vi "DrawOrange.vi"(9 "Expression":string, 11 "String in":refnum<vi>) -> (3 "String out":refnum<vi>)   [LabVIEW 2016, in "Code.xctl"]
uses:
  <userlib>/MicroPython/VIs/ColorText/Code.xctl
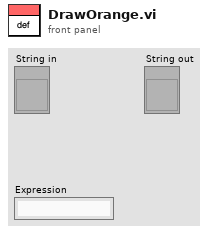
[diagram p1: front panel]
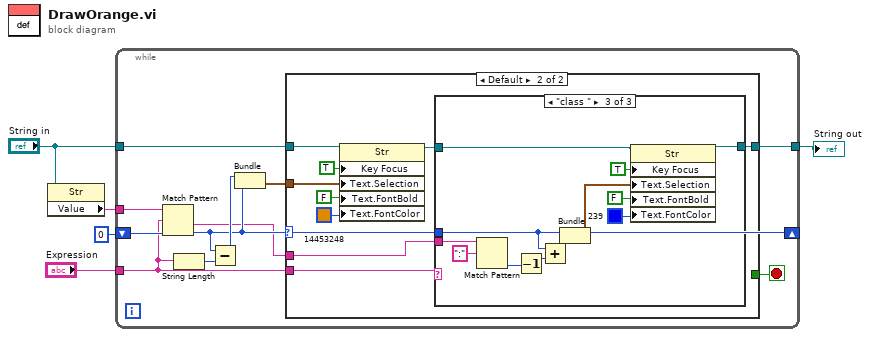
[diagram p0: block diagram]
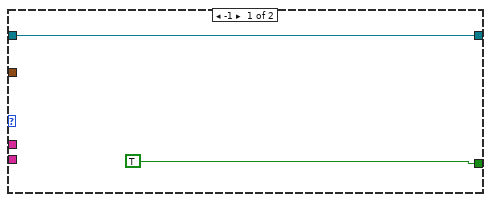
[diagram p2: hidden frame]
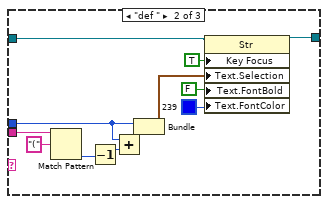
[diagram p4: hidden frame]
diagram:
  n1 = property on="Property Node" class="Str"(reference="String in") -> ("Value"=w1:string)  [unwired: 1 in, 2 out]
  n2 = while {
    tunnel: "String in" -> [w16]
    shift-right: [w9] -> _
    shift-left: 0 -> [w14]
    tunnel: w1 -> [w15]
    tunnel: [w10] -> w4
    tunnel: "Expression" -> [w7]
    stop <- w8 stop-if-true
    n3 = Match Pattern(string=w15, regular expression=w7, offset (0)=w14) -> (after substring=w6:string, offset past match=w9:i32)  [unwired: 2 out]
    n4 = String Length(string=w7) -> (length=w13:i32)
    n5 = Subtract(x=w9, y=w13) -> (x-y=w12:i32)
    n6 = Bundle(w12, "offset past match"=w9) -> (w11:cluster{i32, "offset past match":i32})  [unwired: 1 in]
    n7 = case shown="Default" w9 {
      selector: w9 -> [_ w21]
      tunnel: w16 -> [w18 w25]
      tunnel: w11 -> [_ w24]
      tunnel: [w18 w22] -> w10
      tunnel: [TRUE _] -> w8
      tunnel: w7 -> [_ w20]
      tunnel: w6 -> [_ w19]
      frame -1 {
      }
      frame Default {
        n8 = property on="Property Node" class="Str"(reference=w25, "Key Focus"=TRUE, "Text.Selection"=w24, "Text.FontBold"=FALSE ("Text.Font:Bold"), "Text.FontColor"=u32 14453248 ("Text.Text Colors:Text Color")) -> (reference out=w23:refnum<vi>)  [unwired: 1 in, 1 out]
        n9 = case shown="\"class \"" w20 {
          tunnel: w23 -> [w29 w38 w50]
          tunnel: [w29 w37 w49] -> w22
          tunnel: w21 -> [_ w34 w46]
          tunnel: w19 -> [_ w32 w44]
          frame Default {
          }
          frame "def " {
            n10 = Match Pattern(string=w32, regular expression="(") -> (offset past match=w30:i32)  [unwired: 1 in, 3 out]
            n11 = Decrement(x=w30) -> (x-1=w35:i32)
            n12 = Add(x=w34, y=w35) -> (x+y=w33:i32)
            n13 = Bundle("offset past match"=w34, w33) -> (w36:cluster{"offset past match":i32, i32})  [unwired: 1 in]
            n14 = property on="Property Node" class="Str"(reference=w38, "Key Focus"=TRUE, "Text.Selection"=w36, "Text.FontBold"=FALSE ("Text.Font:Bold"), "Text.FontColor"=u32 239 ("Text.Text Colors:Text Color")) -> (reference out=w37:refnum<vi>)  [unwired: 1 in, 1 out]
          }
          frame "class " {
            n15 = Match Pattern(string=w44, regular expression=":") -> (offset past match=w42:i32)  [unwired: 1 in, 3 out]
            n16 = Decrement(x=w42) -> (x-1=w47:i32)
            n17 = Add(x=w46, y=w47) -> (x+y=w45:i32)
            n18 = Bundle("offset past match"=w46, w45) -> (w48:cluster{"offset past match":i32, i32})  [unwired: 1 in]
            n19 = property on="Property Node" class="Str"(reference=w50, "Key Focus"=TRUE, "Text.Selection"=w48, "Text.FontBold"=FALSE ("Text.Font:Bold"), "Text.FontColor"=u32 239 ("Text.Text Colors:Text Color")) -> (reference out=w49:refnum<vi>)  [unwired: 1 in, 1 out]
          }
        }
      }
    }
  }
  "String out" <- w4
